vi "XIPIN_10G_Ethernet_Subsystem_3_0.vi"   [LabVIEW 2017]
doc: "The IP 10G Ethernet Subsystem provides a 10Gbps Ethernet MAC and PCS/PMA in BASE-R/KR modes, designed to the IEEE802.3 specification. The transmit and receive data interfaces use AXI4-Stream interfaces. An optional AXI4-Lite interface is used for the control interface to internal registers. The core can also provide optional high accuracy IEEE1588-2008 1-step and 2-step hardware time-stamping for BASE-R permutations.\n------------------------------------\n<b>Need License</b> : Yes\n<b>Interface</b> : AXI4 AXI4-Stream"
uses:
  <vilib>/rvi/XilinxIP/XIPIN_XNode/niFpgaXIPIN.xnode
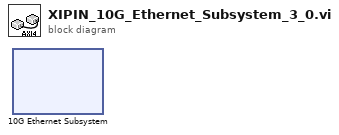
[diagram p0: block diagram]
diagram:
  n1 = xnode ("10G Ethernet Subsystem")() -> ()
